vi "Get App Version.vi"(8 "error in (no error)":errorcluster) -> (0 "error out":errorcluster, 2 "String":string)   [LabVIEW 2023, in "Application.lvlib"]
uses:
  Application.lvlib
  <vilib>/AppBuilder/AB_API_Simple/Get Build Specification Version (path).vi
  <vilib>/AppBuilder/AB_API_Simple/NI_App_Builder_API.lvlib
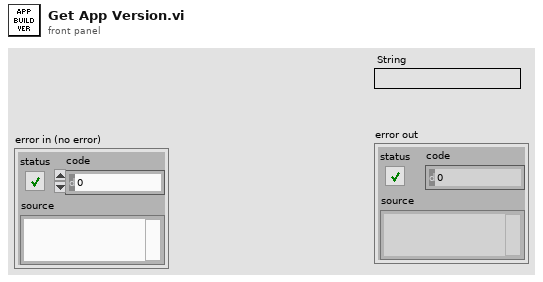
[diagram p1: front panel]
types:
  T1 = enum32{"invalid app kind", "Development System", "Run Time System", "Student Edition", "Embedded LabVIEW", "Evaluation", "Custom"}
  T2 = typedef "NI_App_Builder_API.lvlib/Build Specification Version.ctl" = cluster{"Major":u16, "Minor":u16, "Fix":u16, "Build":u16}
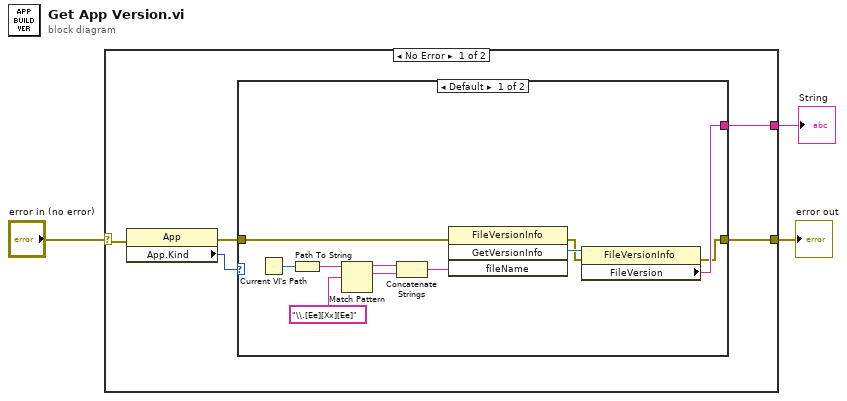
[diagram p0: block diagram]
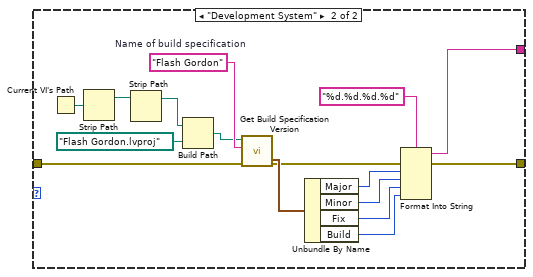
[diagram p2: hidden frame]
diagram:
  n1 = case shown="No Error" "error in (no error)" {
    selector: "error in (no error)" -> [w5 w36]
    tunnel: [w8 w36] -> w3
    tunnel: [w7 _] -> w2
    frame No Error {
      n2 = property class="App"(error in=w5) -> (error out=w6:errorcluster, "App.Kind"=w4:T1)  [unwired: 1 in, 1 out]
      n3 = case shown="Default" w4 {
        tunnel: [w10 w35] -> w8
        tunnel: [w13 w34] -> w7
        tunnel: w6 -> [w12 w32]
        frame Default {
          n4 = Current VI's Path() -> (path=w9:path)
          n5 = Path To String(path=w9) -> (string=w14:string)
          n6 = Match Pattern(string=w14, regular expression="\\.[Ee][Xx][Ee]") -> (before substring=w16:string, match substring=w17:string)  [unwired: 1 in, 2 out]
          n7 = Concatenate Strings(w16, w17) -> (w15:string)
          n8 = invoke class="FileVersionInfo" method="GetVersionInfo"(error in=w12, "fileName"=w15) -> (error out=w11:errorcluster, "GetVersionInfo"=w19:refnum<k24>)  [unwired: 2 in, 2 out]
          n9 = property class="FileVersionInfo"(reference=w19, error in=w11) -> (error out=w10:errorcluster, "FileVersion"=w13:string)  [unwired: 1 out]
        }
        frame "Development System" {
          w25 = "Flash Gordon"  # Name of build specification
          n10 = Current VI's Path() -> (path=w22:path)
          n11 = Strip Path(path=w22) -> (stripped path=w21:path)  [unwired: 1 out]
          n12 = Strip Path(path=w21) -> (stripped path=w20:path)  [unwired: 1 out]
          n13 = Build Path(base path=w20, name or relative path=path "Flash Gordon.lvproj") -> (appended path=w23:path)
          n14 = call-poly <vilib>:"Get Build Specification Version.vi"("error in (no error)"=w32, "Name of build specification"=w25, "Path to project"=w23) -> ("error out"=w26:errorcluster, "Build Specification Version"=w33:T2)  [unwired: 7 in]
          n15 = Unbundle By Name(w33) -> ("Major"=w31:u16, "Minor"=w30:u16, "Fix"=w29:u16, "Build"=w28:u16)
          n16 = Format Into String(format string="%d.%d.%d.%d", error in=w26, w31, w30, w29, w28) -> (resulting string=w34:string, error out=w35:errorcluster)  [unwired: 1 in]
        }
      }
    }
    frame Error {
    }
  }
  "error out" <- w3
  "String" <- w2
